vi "Sample_Finite_WindowTrigger.vi"() -> ()   [LabVIEW 2013]
doc: "This samples demonstrates how to sample a finite waveform."
uses:
  <userlib>/ArtScope/Trigger/ArtScope_ConfigureTriggerWindow.vi
  <userlib>/ArtScope/Fetch/ArtScope_FetchBinary8.vi
  <userlib>/ArtScope/_SubVI/ArtScope_ArrayByChannel_U8.vi
panel:
  in  "reference position":dbl
  in  "window mode":i32(ring) items=["Entering", "Leaving"]
  in  "high level(mV)":dbl=1000.0
  in  "low level(mV)":dbl
  in  "width(ns)":i32
  in  "sensitive(ns)":i32
  in  "count":i32=1
  in  "source":string(combo)="VAL_TRIGGER_ATR"
  in  "range(Vpp)":i32(ring) items=["20V", "10V", "2V", "40V", "16V", "8V", "4V", "1.6V", "800m", "400m", "160m", "80m", "40m"]
  in  "offset(mV)":i32
  in  "num samples":i32=1000
  in  "Stop":bool
  out "waveform":u8[][](graph)
  out "ErrorOutput":errorcluster={"status"=FALSE, "code"=0, "source"="\n"}
  in  "timeout(s)":dbl=10.0
  in  "min record length":i32=6000
  in  "min sample rate":dbl=800000.0
  in  "coupling":i32(ring) items=["DC", "AC"]
  in  "channel name":string="0"
  in  "resource name":string="Dev1"
  # "Vertical"
  # "Horizontal"
  # "Trigger"
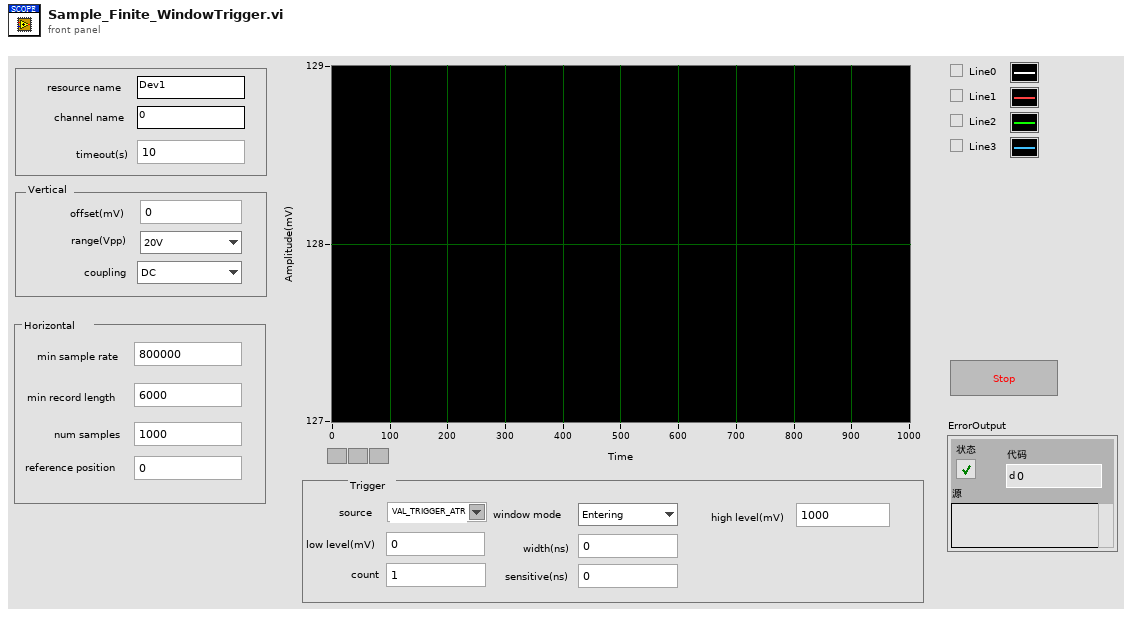
[diagram p1: front panel]
types:
  T1 = cluster{"fLSB":cluster{dbl, dbl, dbl, dbl, dbl, dbl, dbl, dbl}, "RangeValue":cluster{dbl, dbl, dbl, dbl, dbl, dbl, dbl, dbl}, "wMaxLSB":u32, "TriggerMode":i32, "sampLengthPerChan":u32, "pAvailSampsPoints":u32, "channelCount":i32}
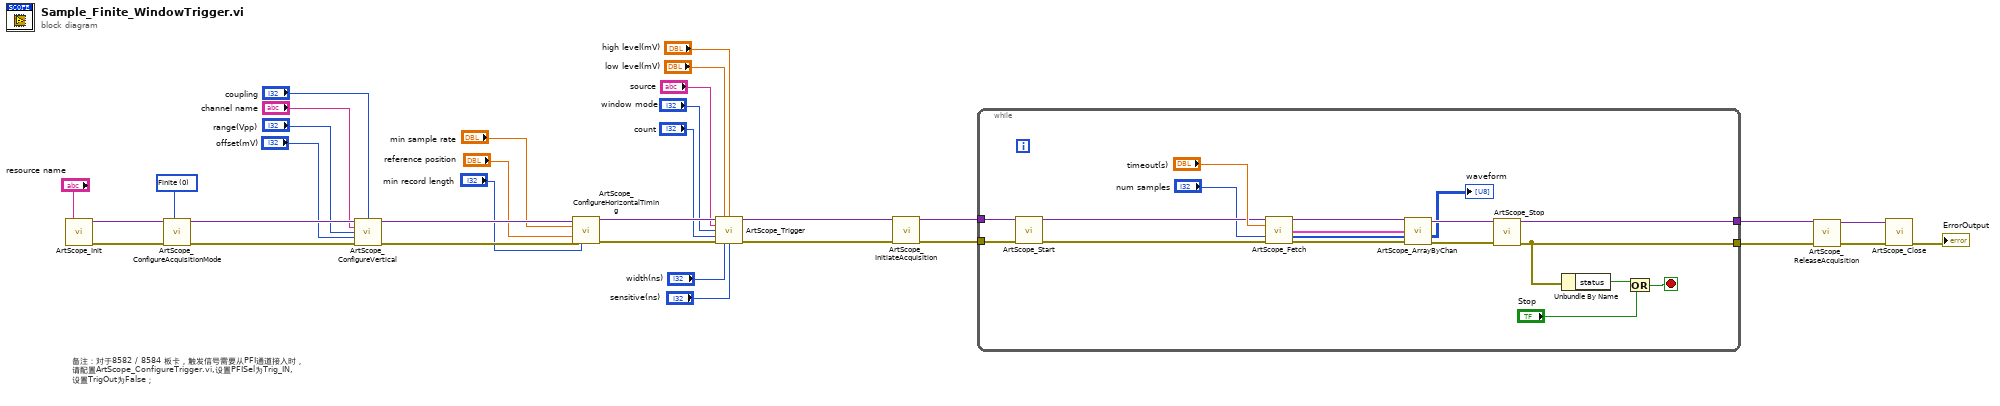
[diagram p0: block diagram]
diagram:
  w25 = 0 items=["Finite", "Continuous"] ("AcuqMode")
  # "备注：对于8582 / 8584 板卡，触发信号需要从PFI通道接入时，\n请配置ArtScope_ConfigureTrigger.vi,设置PFISel为Trig_IN,\n设置TrigOut为False；"
  n1 = call <userlib>:"ArtScope_Init.vi"("task name"="resource name") -> ("task handle"=w26:variant, "error out"=w27:errorcluster)  [unwired: 13 in]
  n2 = call <userlib>:"ArtScope_ConfigureAcquisitionMode.vi"("task handle"=w26, "acquisition mode"=w25, "error in (no error)"=w27) -> ("task handle"=w24:variant, "error out"=w28:errorcluster)  [unwired: 11 in]
  n3 = call <userlib>:"ArtScope_ConfigureVertical.vi"("task handle"=w24, "coupling"="coupling", "channels"="channel name", "range(Vpp)"="range(Vpp)", "offset"="offset(mV)", "error in (no error)"=w28) -> ("task handle"=w31:variant, "error out"=w30:errorcluster)  [unwired: 8 in]
  n4 = call <userlib>:"ArtScope_ConfigureHorizontalTiming.vi"("task handle"=w31, "min sample rate"="min sample rate", "reference position"="reference position", "error in (no error)"=w30, "min record length"="min record length") -> ("task handle"=w22:variant, "error out"=w23:errorcluster)  [unwired: 9 in]
  n5 = call-poly <userlib>:"ArtScope_Trigger.vi"("task handle"=w22, "low level"="low level(mV)", "high level"="high level(mV)", "trigger source"="source", "window mode"="window mode", "trigger count"="count", "error in (no error)"=w23, "trigger coupling"="width(ns)", "trigger sensitive"="sensitive(ns)") -> ("task handle"=w14:variant, "error out"=w13:errorcluster)  [unwired: 5 in]
  n6 = call <userlib>:"ArtScope_InitiateAcquisition.vi"("task handle"=w14, "error in (no error)"=w13) -> ("task handle"=w12:variant, "error out"=w11:errorcluster)  [unwired: 12 in]
  n7 = while {
    tunnel: [w47] -> w18
    tunnel: [w46] -> w17
    tunnel: w12 -> [w45]
    tunnel: w11 -> [w50]
    stop <- w48 stop-if-true
    n8 = call <userlib>:"ArtScope_Start.vi"("task handle"=w45, "error in (no error)"=w50) -> ("task handle"=w43:variant, "error out"=w42:errorcluster)  [unwired: 12 in]
    n9 = call-poly <userlib>:"ArtScope_Fetch.vi"("task handle"=w43, "timeout"="timeout(s)", "num samples"="num samples", "error in (no error)"=w42) -> ("task handle"=w40:variant, "wfm info"=w38:T1, "data"=w37:u8[], "error out"=w39:errorcluster)  [unwired: 8 in]
    n10 = call-poly <userlib>:"ArtScope_ArrayByChan.vi"("task handle"=w40, "wfm info"=w38, "1D data"=w37, "error in (no error)"=w39) -> ("task handle"=w35:variant, "2D data"=→"waveform":u8[][], "error out"=w36:errorcluster)  [unwired: 9 in]
    n11 = call <userlib>:"ArtScope_Stop.vi"("task handle"=w35, "error in (no error)"=w36) -> ("task handle"=w47:variant, "error out"=w46:errorcluster)  [unwired: 12 in]
    n12 = Unbundle By Name(w46) -> ("status"=w49:bool)
    n13 = Or(x=w49, y="Stop") -> (x .or. y?=w48:bool)
  }
  n14 = call <userlib>:"ArtScope_ReleaseAcquisition.vi"("task handle"=w18, "error in (no error)"=w17) -> ("task handle"=w16:variant, "error out"=w15:errorcluster)  [unwired: 12 in]
  n15 = call <userlib>:"ArtScope_Close.vi"("task handle"=w16, "error in (no error)"=w15) -> ("error out"=→"ErrorOutput":errorcluster)  [unwired: 13 in]
